vi "Start.vi"(8 "error in (no error)":errorcluster, 10 "search dirs":path[](array[path]), 11 "comic_crawler in":refnum<class "comic_crawler.lvclass">) -> (0 "error out":errorcluster, 3 "comic_crawler out":refnum<class "comic_crawler.lvclass">)   [LabVIEW 2024, in "comic_crawler.lvclass"]
uses:
  comic_crawler.lvclass
  comic_crawler.lvclass/comic_crawler.ctl
  private/daemon.states--enum.ctl
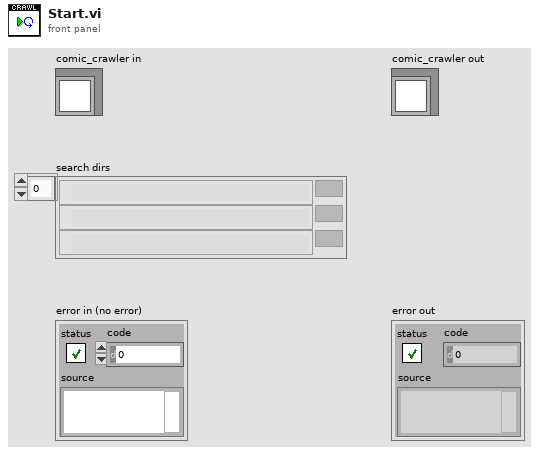
[diagram p1: front panel]
types:
  T1 = typedef "comic_crawler.lvclass/daemon.states--enum.ctl" = enum16{"start search", "idle", "set timer", "running", "stop search", "wait", "set delay", "shut down"}
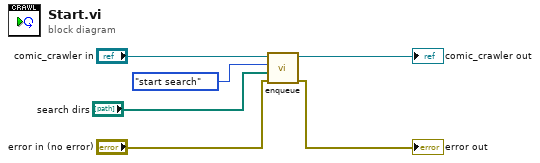
[diagram p0: block diagram]
diagram:
  n1 = call "enqueue.vi"("error in (no error)"="error in (no error)", "data"="search dirs", "cmd"=daemon.states--enum."start search", "comic_crawler in"="comic_crawler in") -> ("error out"=→"error out":errorcluster, "comic_crawler out"=→"comic_crawler out":refnum<class "comic_crawler.lvclass">)  [unwired: 6 in]
